vi "NewCore.vi"(8 "error in (no error)":errorcluster, 10 "ParamsArray":variant[](array[variant]), 11 "Room":refnum<class "Room.lvclass">) -> (0 "error out":errorcluster, 3 "Room":refnum<class "Room.lvclass">)   [LabVIEW 2020, in "Room.lvclass"]
uses:
  Room.lvclass
  Private/TypeDef/privateData.ctl
  MazeSite/MazeSite.lvclass
  TypeDef/RoomParams.ctl
  Room.lvclass/Room.ctl
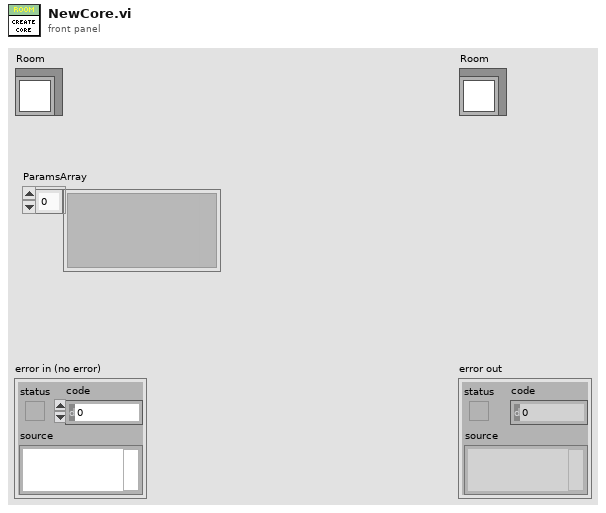
[diagram p1: front panel]
types:
  T1 = typedef "Room.lvclass/RoomParams.ctl" = cluster{"roomNumber":i32}
  T2 = typedef "Room.lvclass/privateData.ctl" = cluster{"sides":refnum<class "MazeSite.lvclass">[], "roomNumber":i32}
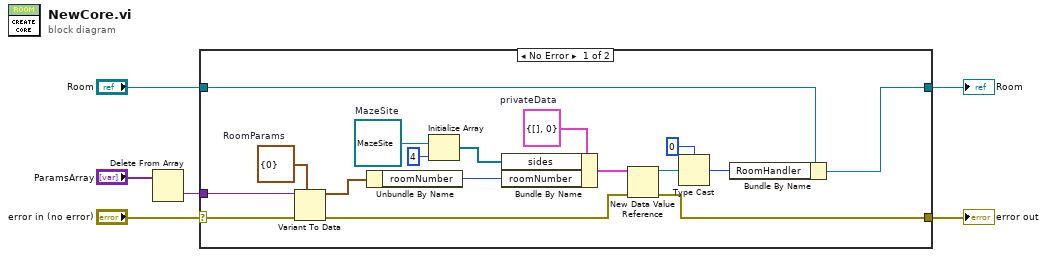
[diagram p0: block diagram]
diagram:
  n1 = Delete From Array(array="ParamsArray") -> (deleted portion=w3:variant)  [unwired: 2 in, 1 out]
  n2 = case shown="No Error" "error in (no error)" {
    selector: "error in (no error)" -> [w12 w25]
    tunnel: [w16 w25] -> w5
    tunnel: [w18 w24] -> w6
    tunnel: "Room" -> [w17 w24]
    tunnel: w3 -> [w10 _]
    frame No Error {
      w8 = refnum<class "MazeSite.lvclass"> refnum  # MazeSite
      w14 = T1 {"roomNumber"=0}  # RoomParams
      w20 = T2 {"sides"=[], "roomNumber"=0}  # privateData
      n3 = Variant To Data(error in=w12, type=w14, Variant=w10) -> (data=w13:T1, error out=w11:errorcluster)
      n4 = Unbundle By Name(w13) -> ("roomNumber"=w15:i32)
      n5 = Initialize Array(w8, 4 ("dimension size")) -> (w7:refnum<class "MazeSite.lvclass">[])
      n6 = Bundle By Name(cluster=w20, "sides"=w7, "roomNumber"=w15) -> (w19:T2)
      n7 = New Data Value Reference(data value=w19, error in=w11) -> (data value reference=w23:refnum<data-value>, error out=w16:errorcluster)
      n8 = Type Cast(type=u32 0, x=w23) -> (*(type *) &x=w21:u32)
      n9 = Bundle By Name(cluster=w17, "RoomHandler"=w21) -> (w18:refnum<class "Room.lvclass">)
    }
    frame Error {
    }
  }
  "error out" <- w5
  "Room" <- w6
